vi "SET_EXT_TRIGG_n.vi"(2 "execute":bool, 7 "EXT_TRIGG":bool, 11 "error in (no error)":errorcluster) -> (4 "function return":string, 15 "error out":errorcluster)   [LabVIEW 2017, in "ZBOX_IS.lvlib"]
uses:
  ZBOX_IS.lvlib
panel:
  out "unsigned 32bit integer":u32
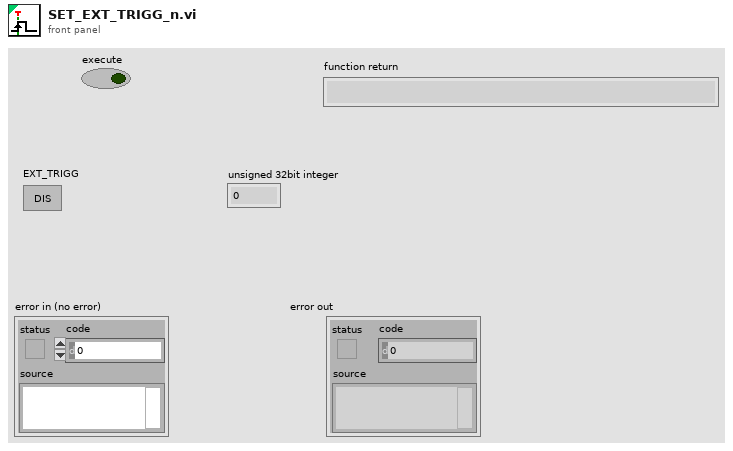
[diagram p1: front panel]
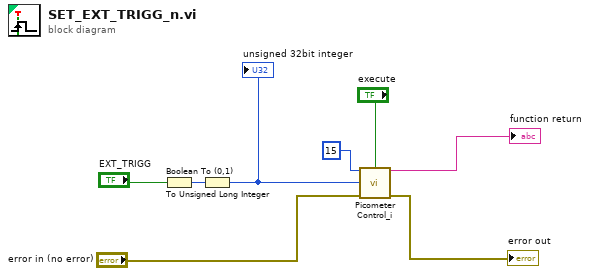
[diagram p0: block diagram]
diagram:
  n1 = Boolean To (0,1)(Boolean="EXT_TRIGG") -> (0, 1=w3:i16)
  n2 = To Unsigned Long Integer(number=w3) -> (unsigned 32bit integer=w2:u32)
  "unsigned 32bit integer" <- w2
  n3 = call "Picometer Control_i.vi"("Cmd"=u8 15, "execute"="execute", "ulValue"=w2, "error in (no error)"="error in (no error)") -> ("function return"=→"function return":string, "error out"=→"error out":errorcluster)  [unwired: 7 in, 3 out]
